vi "Sort Scan Parameters.vi"(2 "Scan parameters":T1=[{"DAQ Channel"=2, "Label"="\nscaledVsg1=", "Start"=0.14, "End"=-0.060000000000000005, "Step"=-0.060000000000000005, "B sweep rate"=0.0}, {"DAQ Channel"=2, "Label"="\nscaledVsg1=", "Start"=0.14, "End"=-0.060000000000000005, "Step"=-0.060000000000000005, "B sweep rate"=0.0}, {"DAQ Channel"=2, "Label"="\nscaledVsg1=", "Start"=0.14, "End"=-0.060000000000000005, "Step"=-0.060000000000000005, "B sweep rate"=0.0}, {"DAQ Channel"=3, "Label"="\nscaledVsg1=", "Start"=0.14, "End"=-0.060000000000000005, "Step"=-0.060000000000000005, "B sweep rate"=0.0}] {"B sweep rate" format="%.2f"; "Step" format="%#_6p"; "End" format="%#_6p"; "Start" format="%#_6p"}, 3 "Scan control":T3=[{"Priority"=enum."Priority 1", "Scan name"=enum."Vsg1"}, {"Priority"=enum."Priority 2", "Scan name"=enum."Vsg2"}, {"Priority"=enum."Priority 0", "Scan name"=enum."Vsgw"}, {"Priority"=enum."Priority 2", "Scan name"=enum."Vbg"}]) -> (0 "Sorted scan parameters":cluster{T1}[](array[cluster])=[{[{"DAQ Channel"=2, "Label"="\nscaledVsg1=", "Start"=0.14, "End"=-0.060000000000000005, "Step"=-0.060000000000000005, "B sweep rate"=0.0}]}, {[{"DAQ Channel"=2, "Label"="\nscaledVsg1=", "Start"=0.14, "End"=-0.060000000000000005, "Step"=-0.060000000000000005, "B sweep rate"=0.0}]}, {[{"DAQ Channel"=2, "Label"="\nscaledVsg1=", "Start"=0.14, "End"=-0.060000000000000005, "Step"=-0.060000000000000005, "B sweep rate"=0.0}, {"DAQ Channel"=3, "Label"="\nscaledVsg1=", "Start"=0.14, "End"=-0.060000000000000005, "Step"=-0.060000000000000005, "B sweep rate"=0.0}]}] {"?"."B sweep rate" format="%.2f"; "?"."Step" format="%#_6p"; "?"."End" format="%#_6p"; "?"."Start" format="%#_6p"}, 1 "Sorted scan control":cluster{T3}[](array[cluster])=[{[{"Priority"=enum."Priority 0", "Scan name"=enum."Vsgw"}]}, {[{"Priority"=enum."Priority 1", "Scan name"=enum."Vsg1"}]}, {[{"Priority"=enum."Priority 2", "Scan name"=enum."Vsg2"}, {"Priority"=enum."Priority 2", "Scan name"=enum."Vbg"}]}])   [LabVIEW 2016]
uses:
  Typedefs/ScanControl.ctl
  Typedefs/Cluster - ScanControl.ctl
  Typedefs/Enum - Priority.ctl
  Typedefs/Enum - Action.ctl
  Typedefs/ScanParamters.ctl
  Typedefs/Cluster - ScanParamters.ctl
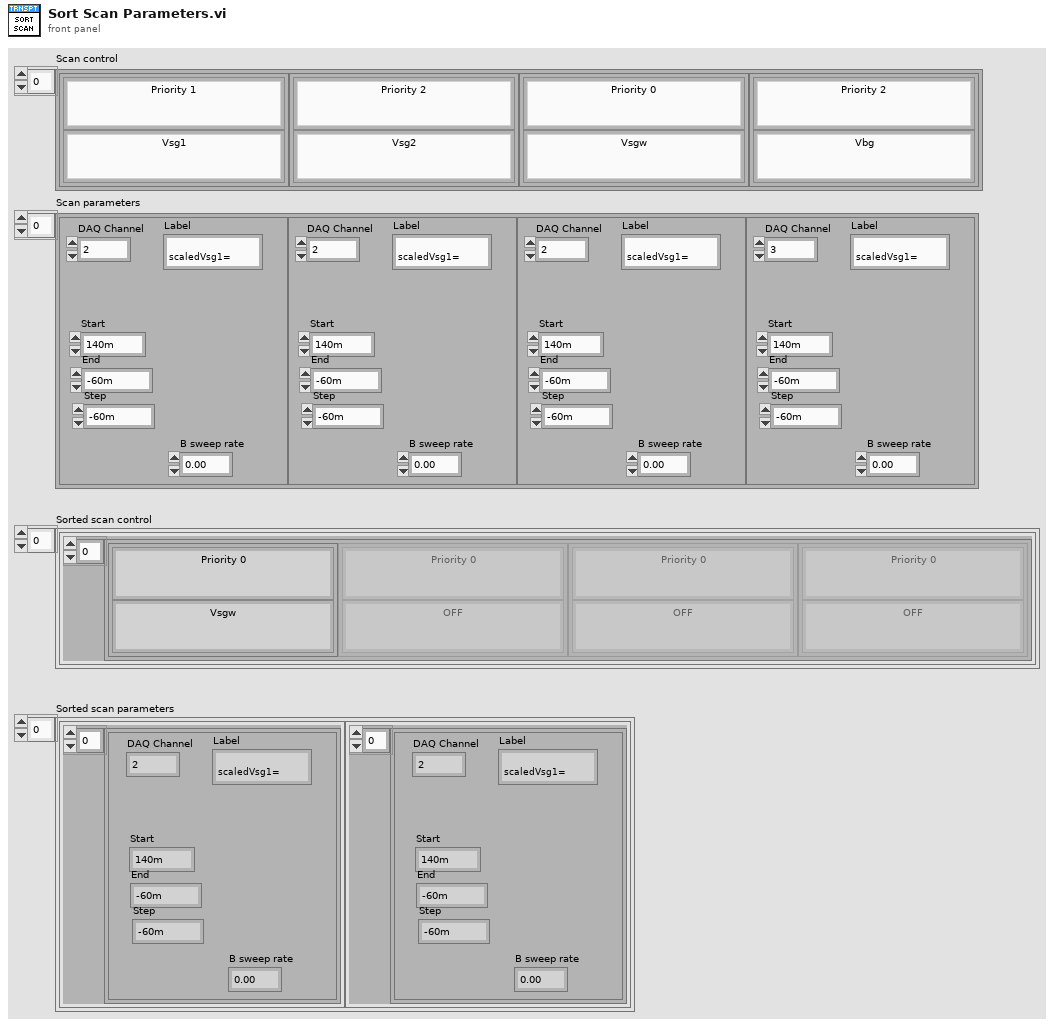
[diagram p1: front panel]
types:
  T1 = typedef "ScanParamters.ctl" = T2[]
  T2 = typedef "Cluster - ScanParamters.ctl" = cluster{"DAQ Channel":i32, "Label":string, "Start":dbl, "End":dbl, "Step":dbl, "B sweep rate":dbl}
  T3 = typedef "ScanControl.ctl" = T4[]
  T4 = typedef "Cluster - ScanControl.ctl" = cluster{"Priority":T5, "Scan name":T6}
  T5 = typedef "Enum - Priority.ctl" = enum16{"Priority 0", "Priority 1", "Priority 2", "Priority 3", "Priority 4", "Priority 5"}
  T6 = typedef "Enum - Action.ctl" = enum16{"OFF", "Vsg1", "Vsg2", "Vsgw", "Vbg", "Vamp", "Field", "Temp", "MW_freq", "MW_amplitude"}
  T7 = cluster{cluster{"DAQ Channel":i32, "Label":string, "Start":dbl, "End":dbl, "Step":dbl, "Step 2":dbl}[]}[]
  T8 = cluster{cluster{"Priority":u16, "Scan name":u16}[]}[]
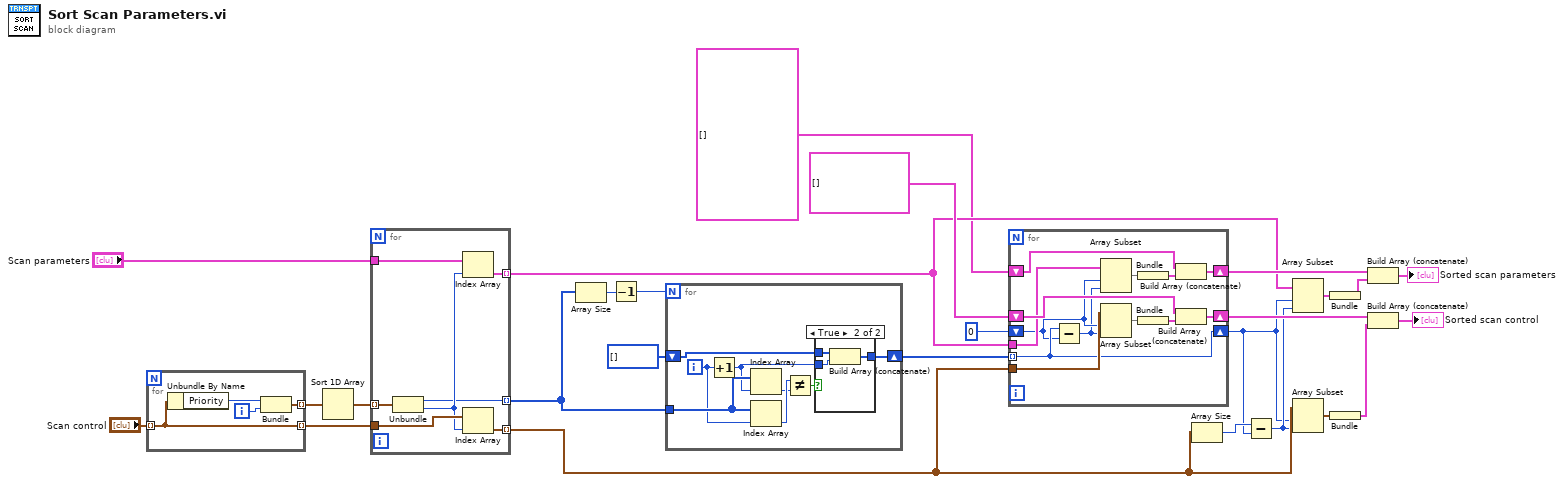
[diagram p0: block diagram]
diagram:
  n1 = for {
    tunnel: "Scan control" -> [w27] mode=indexing
    tunnel: [w30] -> w25 mode=indexing
    tunnel: [w27] -> w23 mode=indexing
    i -> [w28]
    n2 = Unbundle By Name(w27) -> ("Priority"=w29:T5)
    n3 = Bundle("Priority"=w29, w28) -> (w30:cluster{"Priority":T5, i32})  [unwired: 1 in]
  }
  n4 = Sort 1D Array(array=w25) -> (sorted array=w24:cluster{"Priority":T5, i32}[])
  n5 = for {
    tunnel: w24 -> [w37] mode=indexing
    tunnel: w23 -> [w36]
    tunnel: [w35] -> w11 mode=indexing
    tunnel: "Scan parameters" -> [w34]
    tunnel: [w33] -> w6 mode=indexing
    tunnel: [w31] -> w19 mode=indexing
    n6 = Unbundle(w37) -> ("Priority"=w31:T5, w32:i32)
    n7 = Index Array(array=w34, index=w32) -> (element=w33:T2)
    n8 = Index Array(array=w36, index=w32) -> (element=w35:T4)
  }
  n9 = Array Size(array=w19) -> (size(s)=w21:i32)
  n10 = Decrement(x=w21) -> (x-1=w20:i32)
  n11 = for {
    N: w20 -> [_]
    tunnel: w19 -> [w45]
    shift-right: [w41] -> w16
    shift-left: u16[] [] -> [w40]
    i -> [w38]
    n12 = Increment(x=w38) -> (x+1=w39:i32)
    n13 = Index Array(array=w45, index=w39) -> (element=w42:T5)
    n14 = Index Array(array=w45, index=w38) -> (element=w44:T5)
    n15 = Not Equal?(x=w44, y=w42) -> (x != y?=w43:bool)
    n16 = case shown="True" w43 {
      tunnel: [w46 w49] -> w41
      tunnel: w40 -> [w46 w48]
      tunnel: w39 -> [_ w47]
      frame False {
      }
      frame True {
        n17 = Build Array (concatenate)(w48, w47) -> (w49:i32[])
      }
    }
  }
  n18 = for {
    tunnel: w16 -> [w57] mode=indexing
    shift-right: [w62] -> w15
    shift-left: T8 [] -> [w61]
    tunnel: w11 -> [w60]
    shift-right: [w57] -> w4
    shift-left: 0 -> [w55]
    tunnel: w6 -> [w56]
    shift-right: [w52] -> w7
    shift-left: T7 [] -> [w51]
    n19 = Subtract(x=w57, y=w55) -> (x-y=w54:i32)
    n20 = Array Subset(array=w56, index=w55, length=w54) -> (w53:T2[])
    n21 = Array Subset(array=w60, index=w55, length=w54) -> (w59:T4[])
    n22 = Bundle(w53) -> (w50:cluster{T2[]})  [unwired: 1 in]
    n23 = Bundle(w59) -> (w58:cluster{T4[]})  [unwired: 1 in]
    n24 = Build Array (concatenate)(w51, w50) -> (w52:cluster{T2[]}[])
    n25 = Build Array (concatenate)(w61, w58) -> (w62:T8)
  }
  n26 = Array Size(array=w11) -> (size(s)=w12:i32)
  n27 = Subtract(x=w12, y=w4) -> (x-y=w5:i32)
  n28 = Array Subset(array=w6, index=w4, length=w5) -> (w8:T2[])
  n29 = Array Subset(array=w11, index=w4, length=w5) -> (w10:T4[])
  n30 = Bundle(w8) -> (w2:cluster{T2[]})  [unwired: 1 in]
  n31 = Bundle(w10) -> (w9:cluster{T4[]})  [unwired: 1 in]
  n32 = Build Array (concatenate)(w7, w2) -> (→"Sorted scan parameters":cluster{T2[]}[])
  n33 = Build Array (concatenate)(w15, w9) -> (→"Sorted scan control":T8)
